vi "Test-Host-AES-Single-Round-Host.vi"() -> ()   [LabVIEW 2017]
panel:
  out "_a (U32)":u32[](array[numeric]) format="%.0x"
  out "Pass?":bool
  out "exp_c":u32[](array[numeric]) format="%.0x"
  out "act_c":u32[](array[numeric]) format="%.0x"
  out "_c":u32[](array[numeric]) format="%.0x"
  out "_a":u64[](array[numeric]) format="%.0x"
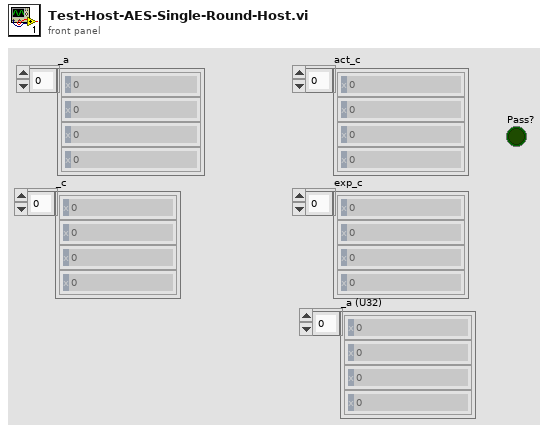
[diagram p1: front panel]
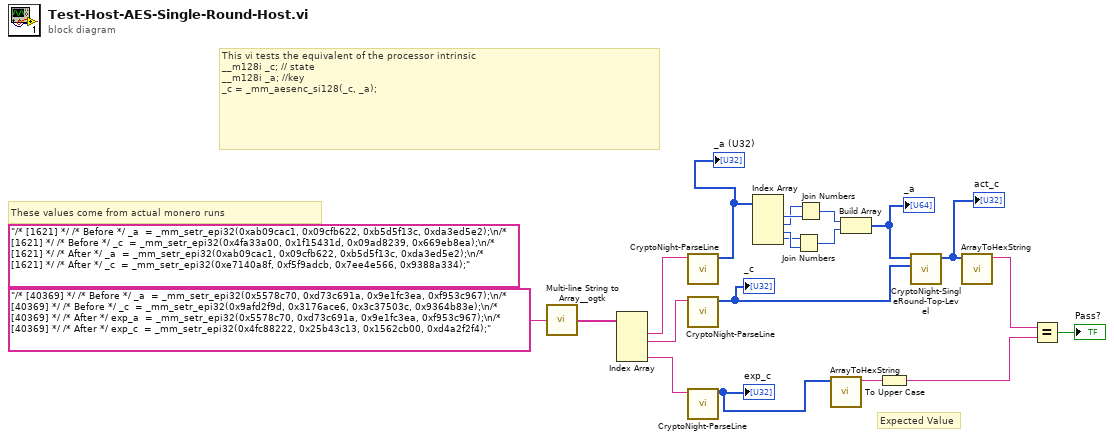
[diagram p0: block diagram]
diagram:
  (unwired) "/* [1621] */ /* Before */ _a  = _mm_setr_epi32(0xab09cac1, 0x09cfb622, 0xb5d5f13c, 0xda3ed5e2);\n/* [1621] */ /* Before */ _c  = _mm_setr_epi32(0x4fa33a00, 0x1f15431d, 0x09ad8239, 0x669eb8ea);\n/* [1621] */ /* After */ _a  = _mm_setr_epi32(0xab09cac1, 0x09cfb622, 0xb5d5f13c, 0xda3ed5e2);\n/* [1621] */ /* After */ _c  = _mm_setr_epi32(0xe7140a8f, 0xf5f9adcb, 0x7ee4e566, 0x9388a334);"
  # "Expected Value"
  # "This vi tests the equivalent of the processor intrinsic\n__m128i _c; // state\n__m128i _a; //key\n_c = _mm_aesenc_si128(_c, _a);"
  # "These values come from actual monero runs"
  n1 = call <userlib>:"Multi-line String to Array__ogtk.vi"("string"="/* [40369] */ /* Before */ _a  = _mm_setr_epi32(0x5578c70, 0xd73c691a, 0x9e1fc3ea, 0xf953c967);\n/* [40369] */ /* Before */ _c  = _mm_setr_epi32(0x9afd2f9d, 0x3176ace6, 0x3c37503c, 0x9364b83e);\n/* [40369] */ /* After */ exp_a  = _mm_setr_epi32(0x5578c70, 0xd73c691a, 0x9e1fc3ea, 0xf953c967);\n/* [40369] */ /* After */ exp_c  = _mm_setr_epi32(0x4fc88222, 0x25b43c13, 0x1562cb00, 0xd4a2f2f4);") -> ("lines"=w17:string[])
  n2 = Index Array(array=w17) -> (element #1=w20:string, element #2=w19:string, element #4=w18:string)  [unwired: 4 in, 1 out]
  n3 = call "CryptoNight-ParseLine.vi"("line"=w20) -> ("Array"=w1:u32[])  [unwired: 10 in]
  "_a (U32)" <- w1
  n4 = call "CryptoNight-ParseLine.vi"("line"=w19) -> ("Array"=w11:u32[])  [unwired: 10 in]
  "_c" <- w11
  n5 = call "CryptoNight-ParseLine.vi"("line"=w18) -> ("Array"=w14:u32[])  [unwired: 10 in]
  "exp_c" <- w14
  n6 = Index Array(array=w1) -> (element #1=w8:u32, element #2=w7:u32, element #3=w6:u32, element #4=w5:u32)  [unwired: 4 in]
  n7 = Join Numbers(hi=w5, lo=w6) -> ((hi.lo)=w4:u64)
  n8 = Join Numbers(hi=w7, lo=w8) -> ((hi.lo)=w3:u64)
  n9 = call "ArrayToHexString.vi"("Array"=w14) -> ("String"=w13:string)  [unwired: 10 in]
  n10 = Build Array(w3, w4) -> (w2:u64[])
  "_a" <- w2
  n11 = To Upper Case(1:w13) -> (0:w15:string)
  n12 = call "CryptoNight-SingleRound-Top-Level.vi"("state (c)"=w11, "key (a)"=w2) -> ("state out (c)"=w9:u32[])  [unwired: 9 in]
  "act_c" <- w9
  n13 = call "ArrayToHexString.vi"("Array"=w9) -> ("String"=w12:string)  [unwired: 10 in]
  n14 = Equal?(x=w12, y=w15) -> (x = y?=→"Pass?":bool)
